vi "Senden.vi"(0 "FPGA VI Reference In":refnum<k20>, 1 "BefehlsCluster":T1, 2 "Senden?":bool[](array[boolean]), 3 "Abfragenr.Cluster":cluster{i32, i32, i32}, 5 "AbfragenCluster":cluster{string[], string[], string[]}) -> (6 "Senden?":bool[](array[boolean]), 7 "Abfragenr.Cluster":cluster{i32, i32, i32}, 8 "BefehlsCluster":T1)   [LabVIEW 2010]
uses:
  <vilib>/rvi/interface/nirviMethod/nirviMethod.xnode
  C:/Users/HAGAR-IV/Desktop/Zeugs/markus/version feb 2012/FPGA Bitfiles/pertrasgcfpga2_FPGATarget_FPGA-Programm-10_16368CB6.lvbitx
  C:/Users/HAGAR-IV/Desktop/Zeugs/Johnny/pertrasgc fpga/FPGA-Programm-10-14.vi
  <vilib>/rvi/interface/common/niFpgaNodeNameForErrorReporting.ctl
  <vilib>/rvi/errors/niLvFpgaWhatHappensToTopLevelVI.ctl
  <vilib>/Utility/error.llb/Error Cluster From Error Code.vi
  <vilib>/rvi/errors/niLvFpgaAdjustHostInterfaceError.vi
  NiFpgaLv.dll
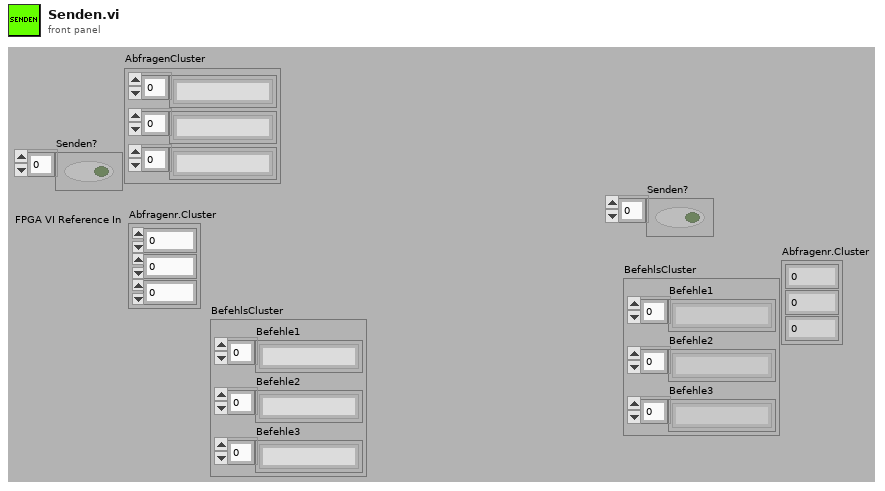
[diagram p1: front panel]
types:
  T1 = cluster{"Befehle1":string[], "Befehle2":string[], "Befehle3":string[]}
  T2 = typedef "niFpgaNodeNameForErrorReporting.ctl" = enum16{"Open FPGA VI Reference", "Read/Write Control", "Invoke Method: Abort", "Invoke Method: Acknowledge IRQ", "Invoke Method: Download", "Invoke Method: FIFO.Configure", "Invoke Method: FIFO.Read", "Invoke Method: FIFO.Start", "Invoke Method: FIFO.Stop", "Invoke Method: FIFO.Write", "Invoke Method: Reset", "Invoke Method: Run", "Invoke Method: Wait on IRQ", "Close FPGA VI Reference"}
  T3 = typedef "niLvFpgaWhatHappensToTopLevelVI.ctl" = enum16{"top level VI scripted behind XNode", "top level VI inlined behind XNode"}
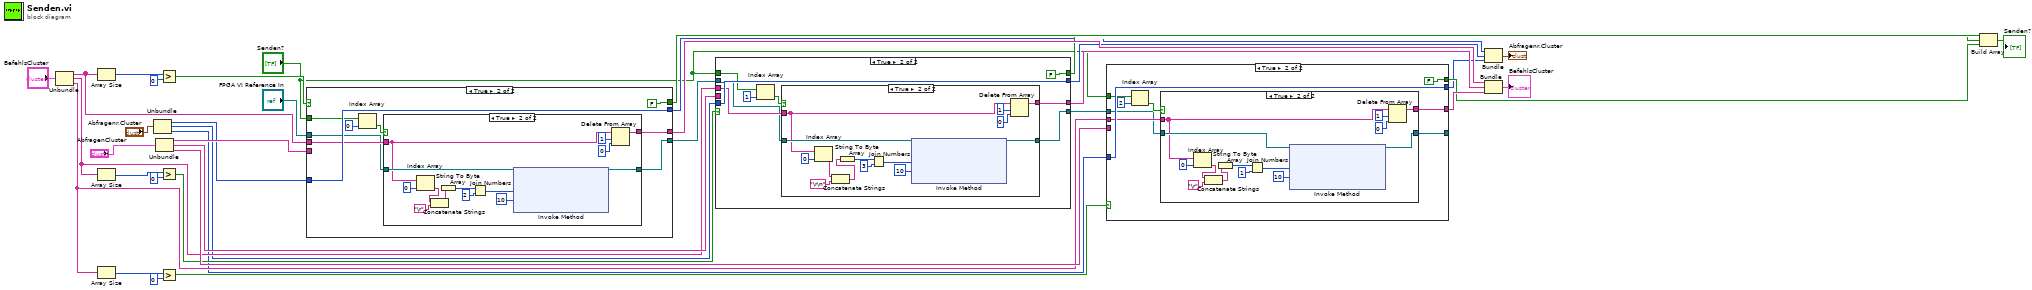
[diagram p0: block diagram]
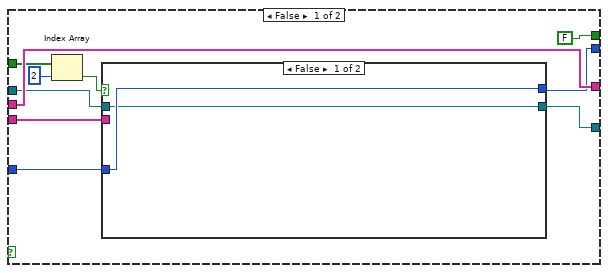
[diagram p2: hidden frame]
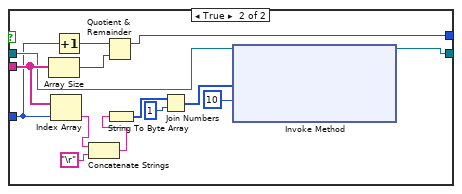
[diagram p3: hidden frame]
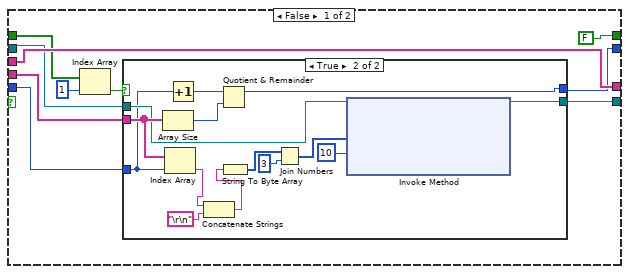
[diagram p5: hidden frame]
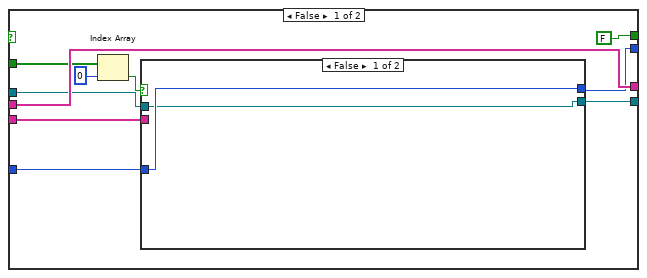
[diagram p8: hidden frame]
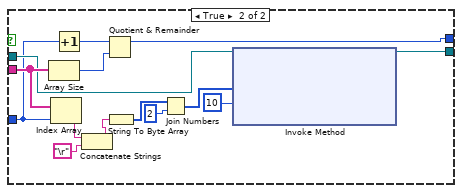
[diagram p9: hidden frame]
diagram:
  n1 = Unbundle("BefehlsCluster") -> ("Befehle1"=w21:string[], "Befehle2"=w20:string[], "Befehle3"=w19:string[])
  n2 = Array Size(array=w21) -> (size(s)=w36:i32)
  n3 = Array Size(array=w20) -> (size(s)=w30:i32)
  n4 = Array Size(array=w19) -> (size(s)=w27:i32)
  n5 = Unbundle("Abfragenr.Cluster") -> (w9:i32, w8:i32, w7:i32)
  n6 = Unbundle("AbfragenCluster") -> (w33:string[], w32:string[], w31:string[])
  n7 = Greater?(x=w36, y=0) -> (0:w34:bool)
  n8 = Greater?(x=w30, y=0) -> (0:w28:bool)
  n9 = Greater?(x=w27, y=0) -> (0:w25:bool)
  n10 = case shown="True" w34 {
    tunnel: w21 -> [w47 w135]
    tunnel: [w47 w134] -> w18
    tunnel: "Senden?" -> [w41 w132]
    tunnel: [FALSE FALSE] -> w14
    tunnel: w9 -> [w44 w138]
    tunnel: "FPGA VI Reference In" -> [w43 w133]
    tunnel: [w42 w138] -> w6
    tunnel: w33 -> [w40 _]
    tunnel: [w39 w131] -> w24
    frame False {
      n11 = Index Array(array=w41, index=0 ("Index")) -> (element=w45:bool)
      n12 = case shown="False" w45 {
        tunnel: w40 -> [_ w61]
        tunnel: w44 -> [w49 w55]
        tunnel: w43 -> [w48 w58]
        tunnel: [w49 w54] -> w42
        tunnel: [w48 w53] -> w39
        frame False {
        }
        frame True {
          n13 = Array Size(array=w61) -> (size(s)=w62:i32)
          n14 = Index Array(array=w61, index=w55) -> (element=w51:string)
          n15 = Increment(x=w55) -> (x+1=w63:i32)
          n16 = Concatenate Strings(w51, "\r") -> (w52:string)
          n17 = Quotient & Remainder(x=w63, y=w62) -> (x-y*floor(x/y)=w54:i32)  [unwired: 1 out]
          n18 = String To Byte Array(string=w52) -> (unsigned byte array=w60:u8[])
          n19 = Join Numbers(hi=w60, lo=u8 2) -> ((hi.lo)=w57:u16[])
          n20 = xnode "Invoke Method"("FPGA VI Reference In"=w58, "Data"=w57, "Timeout (ms)"=10) -> ("FPGA VI Reference Out"=w53:refnum<k20>)  [unwired: 1 in, 2 out]
        }
      }
    }
    frame True {
      n21 = Index Array(array=w132, index=0 ("Index")) -> (element=w136:bool)
      n22 = case shown="True" w136 {
        tunnel: w135 -> [w140 w150]
        tunnel: [w140 w152] -> w134
        tunnel: w133 -> [w139 w151]
        tunnel: [w139 w144] -> w131
        frame False {
        }
        frame True {
          n23 = Index Array(array=w150, index=0 ("Index")) -> (element=w142:string)
          n24 = Concatenate Strings(w142, "\r") -> (w141:string)
          n25 = String To Byte Array(string=w141) -> (unsigned byte array=w148:u8[])
          n26 = Join Numbers(hi=w148, lo=u8 2) -> ((hi.lo)=w146:u16[])
          n27 = xnode "Invoke Method"("FPGA VI Reference In"=w151, "Data"=w146, "Timeout (ms)"=10) -> ("FPGA VI Reference Out"=w144:refnum<k20>)  [unwired: 1 in, 2 out]
          n28 = Delete From Array(array=w150, length=1 ("Länge"), index=0 ("Index")) -> (array with subset deleted=w152:string[])  [unwired: 1 out]
        }
      }
    }
  }
  n29 = case shown="True" w28 {
    tunnel: w20 -> [w230 w318]
    tunnel: [w230 w317] -> w17
    tunnel: "Senden?" -> [w224 w315]
    tunnel: w8 -> [w227 w321]
    tunnel: w24 -> [w226 w316]
    tunnel: [w225 w321] -> w5
    tunnel: w32 -> [w223 _]
    tunnel: [w222 w314] -> w23
    tunnel: [FALSE FALSE] -> w12
    frame False {
      n30 = Index Array(array=w224, index=1 ("Index")) -> (element=w228:bool)
      n31 = case shown="True" w228 {
        tunnel: w223 -> [_ w244]
        tunnel: w227 -> [w232 w238]
        tunnel: w226 -> [w231 w241]
        tunnel: [w232 w237] -> w225
        tunnel: [w231 w236] -> w222
        frame False {
        }
        frame True {
          n32 = Array Size(array=w244) -> (size(s)=w245:i32)
          n33 = Index Array(array=w244, index=w238) -> (element=w234:string)
          n34 = Increment(x=w238) -> (x+1=w246:i32)
          n35 = Concatenate Strings(w234, "\r\n") -> (w233:string)
          n36 = Quotient & Remainder(x=w246, y=w245) -> (x-y*floor(x/y)=w237:i32)  [unwired: 1 out]
          n37 = String To Byte Array(string=w233) -> (unsigned byte array=w243:u8[])
          n38 = Join Numbers(hi=w243, lo=u8 3) -> ((hi.lo)=w240:u16[])
          n39 = xnode "Invoke Method"("FPGA VI Reference In"=w241, "Data"=w240, "Timeout (ms)"=10) -> ("FPGA VI Reference Out"=w236:refnum<k20>)  [unwired: 1 in, 2 out]
        }
      }
    }
    frame True {
      n40 = Index Array(array=w315, index=1 ("Index")) -> (element=w319:bool)
      n41 = case shown="True" w319 {
        tunnel: w318 -> [w323 w333]
        tunnel: [w323 w335] -> w317
        tunnel: w316 -> [w322 w334]
        tunnel: [w322 w327] -> w314
        frame False {
        }
        frame True {
          n42 = Index Array(array=w333, index=0 ("Index")) -> (element=w325:string)
          n43 = Concatenate Strings(w325, "\r\n") -> (w324:string)
          n44 = String To Byte Array(string=w324) -> (unsigned byte array=w331:u8[])
          n45 = Join Numbers(hi=w331, lo=u8 3) -> ((hi.lo)=w329:u16[])
          n46 = xnode "Invoke Method"("FPGA VI Reference In"=w334, "Data"=w329, "Timeout (ms)"=10) -> ("FPGA VI Reference Out"=w327:refnum<k20>)  [unwired: 1 in, 2 out]
          n47 = Delete From Array(array=w333, length=1 ("Länge"), index=0 ("Index")) -> (array with subset deleted=w335:string[])  [unwired: 1 out]
        }
      }
    }
  }
  n48 = case shown="True" w25 {
    tunnel: w19 -> [w413 w501]
    tunnel: [w413 w500] -> w16
    tunnel: "Senden?" -> [w407 w498]
    tunnel: w7 -> [w410 w504]
    tunnel: w23 -> [w409 w499]
    tunnel: [w408 w504] -> w4
    tunnel: w31 -> [w406 _]
    tunnel: [FALSE FALSE] -> w11
    tunnel: [w404 w496] -> _
    frame False {
      n49 = Index Array(array=w407, index=2 ("Index")) -> (element=w411:bool)
      n50 = case shown="False" w411 {
        tunnel: w406 -> [_ w427]
        tunnel: w410 -> [w415 w421]
        tunnel: w409 -> [w414 w424]
        tunnel: [w415 w420] -> w408
        tunnel: [w414 w419] -> w404
        frame False {
        }
        frame True {
          n51 = Array Size(array=w427) -> (size(s)=w428:i32)
          n52 = Index Array(array=w427, index=w421) -> (element=w417:string)
          n53 = Increment(x=w421) -> (x+1=w429:i32)
          n54 = Concatenate Strings(w417, "\r") -> (w416:string)
          n55 = Quotient & Remainder(x=w429, y=w428) -> (x-y*floor(x/y)=w420:i32)  [unwired: 1 out]
          n56 = String To Byte Array(string=w416) -> (unsigned byte array=w426:u8[])
          n57 = Join Numbers(hi=w426, lo=u8 1) -> ((hi.lo)=w423:u16[])
          n58 = xnode "Invoke Method"("FPGA VI Reference In"=w424, "Data"=w423, "Timeout (ms)"=10) -> ("FPGA VI Reference Out"=w419:refnum<k20>)  [unwired: 1 in, 2 out]
        }
      }
    }
    frame True {
      n59 = Index Array(array=w498, index=2 ("Index")) -> (element=w502:bool)
      n60 = case shown="True" w502 {
        tunnel: w501 -> [w506 w516]
        tunnel: [w506 w518] -> w500
        tunnel: w499 -> [w505 w517]
        tunnel: [w505 w510] -> w496
        frame False {
        }
        frame True {
          n61 = Index Array(array=w516, index=0 ("Index")) -> (element=w508:string)
          n62 = Concatenate Strings(w508, "\r") -> (w507:string)
          n63 = String To Byte Array(string=w507) -> (unsigned byte array=w514:u8[])
          n64 = Join Numbers(hi=w514, lo=u8 1) -> ((hi.lo)=w512:u16[])
          n65 = xnode "Invoke Method"("FPGA VI Reference In"=w517, "Data"=w512, "Timeout (ms)"=10) -> ("FPGA VI Reference Out"=w510:refnum<k20>)  [unwired: 1 in, 2 out]
          n66 = Delete From Array(array=w516, length=1 ("Länge"), index=0 ("Index")) -> (array with subset deleted=w518:string[])  [unwired: 1 out]
        }
      }
    }
  }
  n67 = Bundle(w6, w5, w4) -> (→"Abfragenr.Cluster":cluster{i32, i32, i32})  [unwired: 1 in]
  n68 = Bundle("Befehle1"=w18, "Befehle2"=w17, "Befehle3"=w16) -> (→"BefehlsCluster":T1)  [unwired: 1 in]
  n69 = Build Array(w14, w12, w11) -> (→"Senden?":bool[])
